vi "Handle.vi"(8 "error in (no error)":errorcluster, 11 "PublisherGS in":refnum<class "PublisherGS.lvclass">) -> (0 "error out":errorcluster, 3 "PublisherGS out":refnum<class "PublisherGS.lvclass">)   [LabVIEW 2018, in "PublisherGS.lvclass"]
uses:
  PublisherGS.lvclass
  PublisherGS.lvclass/PublisherGS.ctl
  Client/Client.lvclass
  Comm/Stream/Stream.lvclass
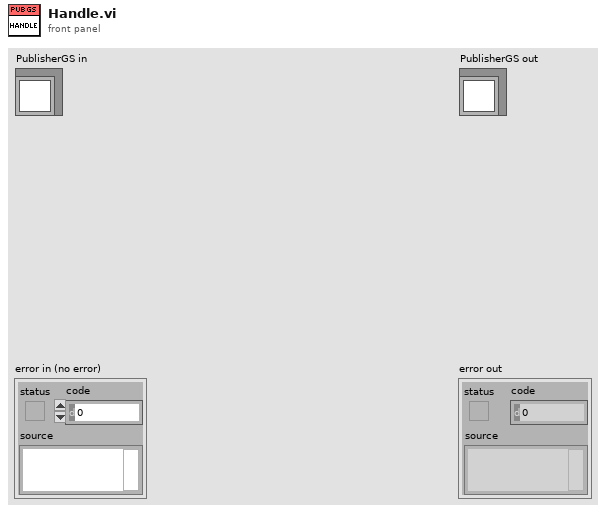
[diagram p1: front panel]
types:
  T1 = cluster{"FocusPhot":dbl, "FocusPolar":dbl, "FocusEffic":dbl, "FocusInstrum":dbl, "ICS":bool, "AG":bool, "broker":string, "timestamp":string}
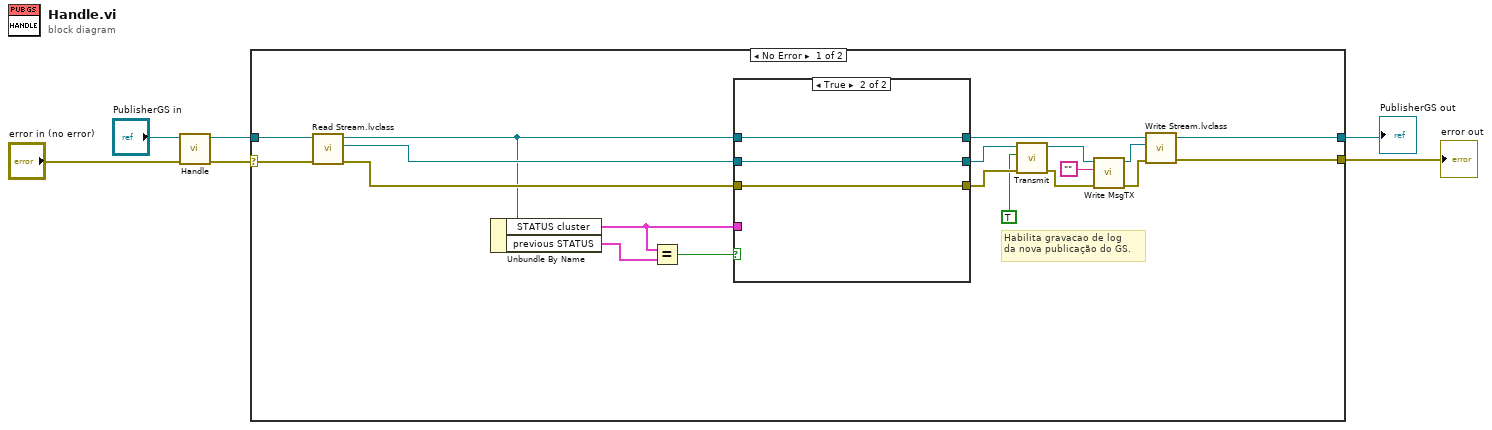
[diagram p0: block diagram]
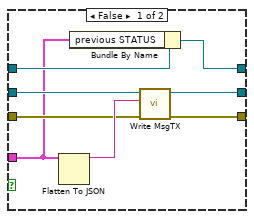
[diagram p2: hidden frame]
diagram:
  n1 = call-parent "Handle.vi"("error in (no error)"="error in (no error)", "Client in"="PublisherGS in") -> ("error out"=w3:errorcluster, "Client out"=w4:refnum<class "PublisherGS.lvclass">)  [unwired: 8 in]
  n2 = case shown="No Error" w3 {
    selector: w3 -> [w24 w38]
    tunnel: [w19 w38] -> w2
    tunnel: [w20 w37] -> w1
    tunnel: w4 -> [w25 w37]
    frame No Error {
      # "Habilita gravacao de log\nda nova publicação do GS."
      n3 = call-dynamic "Read Stream.lvclass.vi"("error in (no error)"=w24, "Client in"=w25) -> ("error out"=w18:errorcluster, "Stream.lvclass"=w21:refnum<class "Stream.lvclass">, "Client out"=w10:refnum<class "PublisherGS.lvclass">)  [unwired: 7 in]
      n4 = Unbundle By Name(w10) -> ("STATUS cluster"=w11:T1, "previous STATUS"=w17:T1)
      n5 = Equal?(x=w11, y=w17) -> (x = y?=w8:bool)
      n6 = case shown="True" w8 {
        tunnel: [w33 w36] -> w23
        tunnel: [w32 w35] -> w22
        tunnel: w21 -> [w31 w36]
        tunnel: w18 -> [w29 w35]
        tunnel: w11 -> [w27 _]
        tunnel: [w26 w34] -> w9
        tunnel: w10 -> [w28 w34]
        frame False {
          n7 = Flatten To JSON(anything=w27) -> (JSON string=w30:string)  [unwired: 2 in, 1 out]
          n8 = Bundle By Name(cluster=w28, "previous STATUS"=w27) -> (w26:refnum<class "PublisherGS.lvclass">)
          n9 = call-dynamic "Write MsgTX.vi"("error in (no error)"=w29, "MsgTX"=w30, "Comm in"=w31) -> ("error out"=w32:errorcluster, "Comm out"=w33:refnum<class "Stream.lvclass">)  [unwired: 7 in]
        }
        frame True {
        }
      }
      n10 = call-dynamic "Transmit.vi"("error in (no error)"=w22, "log?"=TRUE, "Stream in"=w23) -> ("error out"=w15:errorcluster, "Stream out"=w16:refnum<class "Stream.lvclass">)  [unwired: 7 in]
      n11 = call-dynamic "Write MsgTX.vi"("error in (no error)"=w15, "MsgTX"="", "Comm in"=w16) -> ("error out"=w14:errorcluster, "Comm out"=w13:refnum<class "Stream.lvclass">)  [unwired: 7 in]
      n12 = call-dynamic "Write Stream.lvclass.vi"("error in (no error)"=w14, "Stream.lvclass"=w13, "Client in"=w9) -> ("error out"=w19:errorcluster, "Client out"=w20:refnum<class "PublisherGS.lvclass">)  [unwired: 7 in]
    }
    frame Error {
    }
  }
  "error out" <- w2
  "PublisherGS out" <- w1
